vi "Read from File.vi"(7 "Section Name":string, 8 "error in (no error)":errorcluster, 10 "INI Ref":T1, 11 "Image Assertion in":refnum<class "Image Assertion.lvclass">) -> (0 "error out":errorcluster, 2 "INI Ref out":T1, 3 "Image Assertion out":refnum<class "Image Assertion.lvclass">)   [LabVIEW 2020, in "MacroAssert.lvlib" / "Image Assertion.lvclass"]
doc: "Reads associated parameters from the file identified by <B>INI Ref</B>."
uses:
  Image Assertion.lvclass
  <vilib>/Utility/config.llb/Config Data RefNum.ctl
  Image Assertion Type.ctl
  Image Comparator.ctl
  Image Units.ctl
  Compare Method.ctl
  <vilib>/picture/picture.llb/imagedata.ctl
  <vilib>/Utility/error.llb/Error Cluster From Error Code.vi
  <vilib>/Utility/config.llb/Read Key (String).vi
  <vilib>/Utility/config.llb/Read Key (I32).vi
  <vilib>/Utility/config.llb/Read Key (Double).vi
  Assertion Step/Assertion Step.lvclass
  SubVIs/Custom Errors/Custom Errors.lvlib
  <vilib>/Utility/config.llb/NI_LVConfig.lvlib
  MacroAssert.lvlib
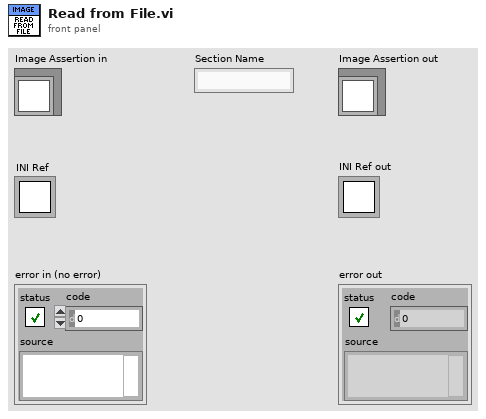
[diagram p1: front panel]
types:
  T1 = typedef "NI_LVConfig.lvlib/Config Data RefNum.ctl" = refnum<k1>
  T2 = typedef "MacroAssert.lvlib/Image Assertion.lvclass/Image Assertion Type.ctl" = enum16{"Control Image", "VI Image", "Window Image", "Cursor Icon"}
  T3 = typedef "MacroAssert.lvlib/Image Assertion.lvclass/Image Comparator.ctl" = enum16{"Is less than or equal to", "Is greater than or equal to"}
  T4 = typedef "MacroAssert.lvlib/Image Assertion.lvclass/Image Units.ctl" = enum16{"Pixels", "Percent"}
  T5 = typedef "MacroAssert.lvlib/Image Assertion.lvclass/Compare Method.ctl" = enum16{"Mean Squared Error", "Peak Signal-to-Noise Ratio"}
  T6 = typedef "imagedata.ctl" = cluster{"image type":i32, "image depth":i32, "image":u8[], "mask":u8[], "colors":u32[], "Rectangle":cluster{"left":i16, "top":i16, "right":i16, "bottom":i16}}
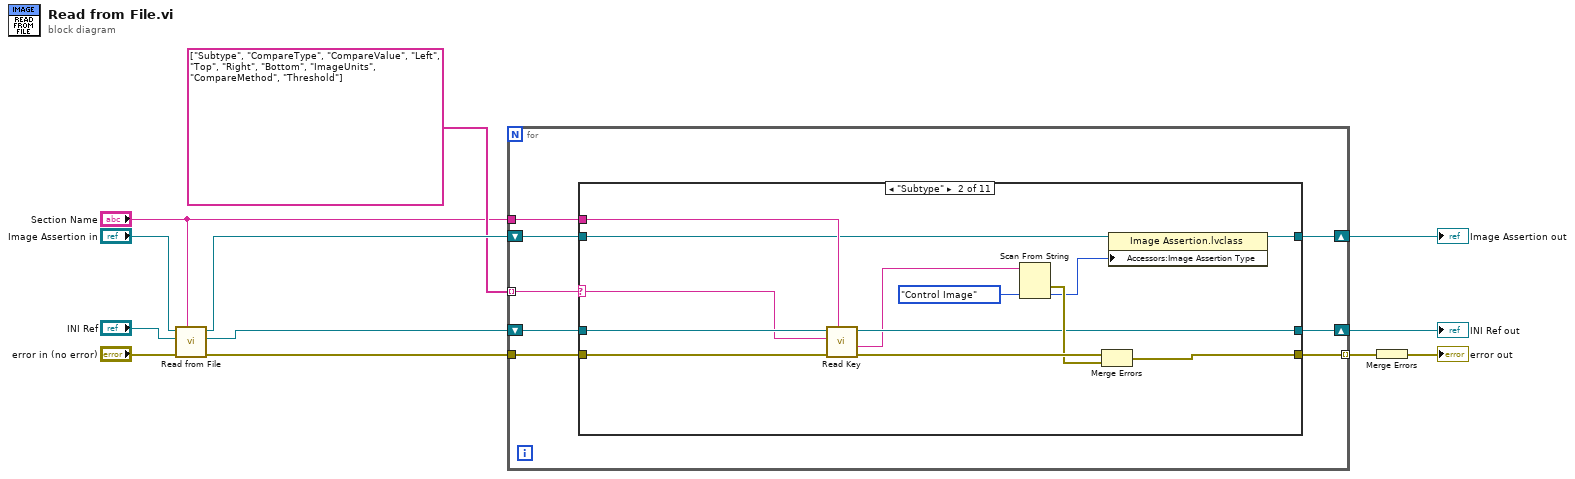
[diagram p0: block diagram]
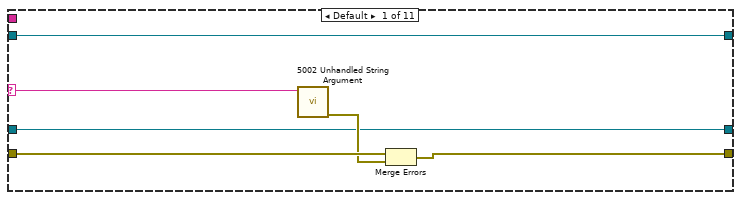
[diagram p2: hidden frame]
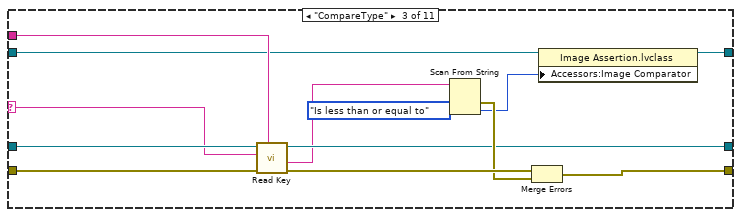
[diagram p3: hidden frame]
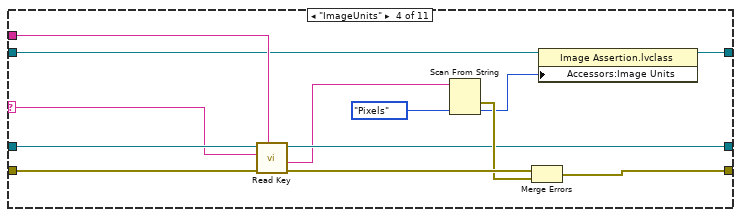
[diagram p4: hidden frame]
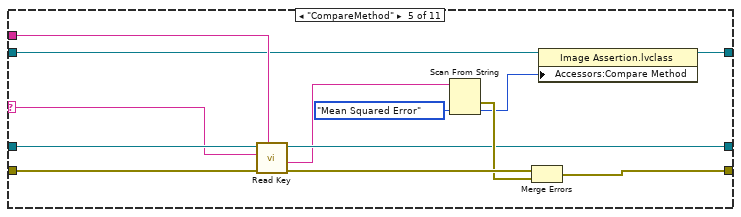
[diagram p5: hidden frame]
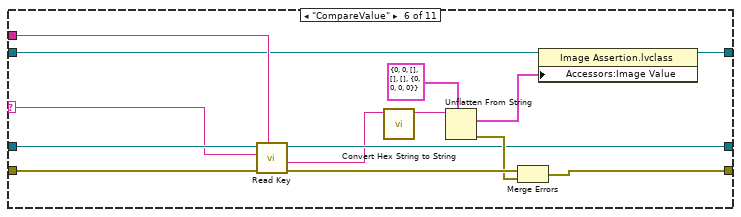
[diagram p6: hidden frame]
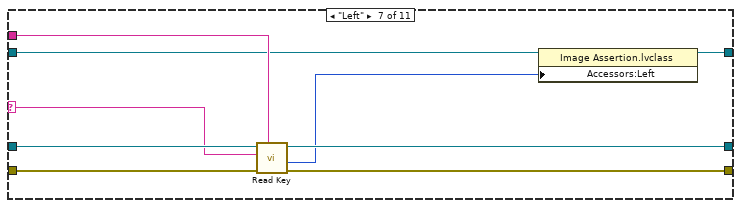
[diagram p7: hidden frame]
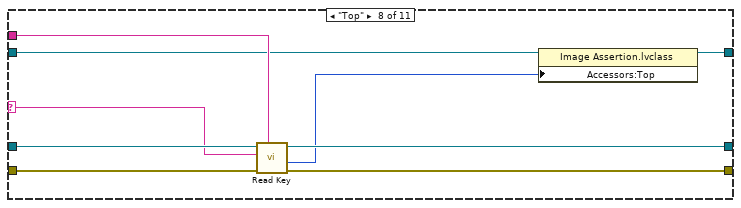
[diagram p8: hidden frame]
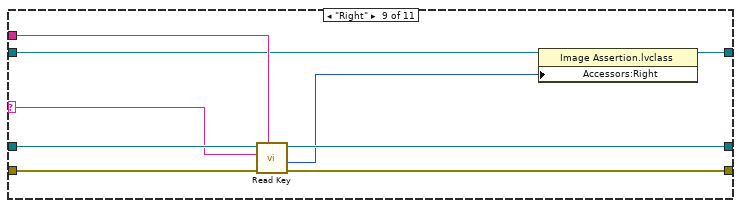
[diagram p9: hidden frame]
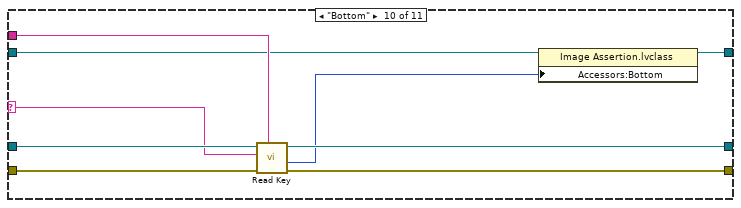
[diagram p10: hidden frame]
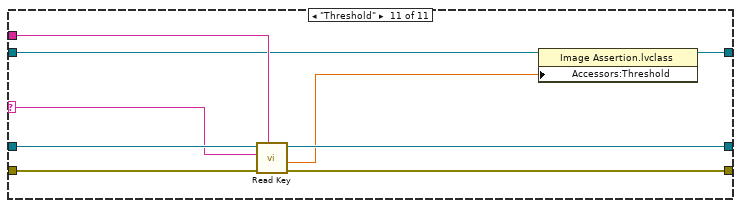
[diagram p11: hidden frame]
diagram:
  n1 = call-parent "Read from File.vi"("Section Name"="Section Name", "error in (no error)"="error in (no error)", "INI Ref"="INI Ref", "Assertion Step in"="Image Assertion in") -> ("error out"=w12:errorcluster, "INI Ref out"=w9:T1, "Assertion Step out"=w6:refnum<class "Image Assertion.lvclass">)  [unwired: 5 in]
  n2 = for {
    tunnel: string[] ["Subtype", "CompareType", "CompareValue", "Left", "Top", "Right", "Bottom", "ImageUnits", "CompareMethod", "Threshold"] -> [w16] mode=indexing
    tunnel: w12 -> [w20]
    tunnel: "Section Name" -> [w15]
    shift-right: [w13] -> w2
    shift-left: w6 -> [w14]
    tunnel: [w19] -> w4 mode=indexing
    shift-right: [w17] -> w7
    shift-left: w9 -> [w18]
    n3 = case shown="\"Subtype\"" w16 {
      selector: w16 -> [w21 w30 w43 w56 w69 w83 w94 w103 w112 w121 w130]
      tunnel: w20 -> [w26 w39 w52 w65 w78 w92 w101 w110 w119 w128 w137]
      tunnel: w15 -> [_ w33 w46 w59 w72 w86 w97 w106 w115 w124 w133]
      tunnel: w14 -> [w22 w32 w45 w58 w71 w85 w96 w105 w114 w123 w132]
      tunnel: [w22 w31 w44 w57 w70 w84 w95 w104 w113 w122 w131] -> w13
      tunnel: [w24 w37 w50 w63 w76 w89 w100 w109 w118 w127 w136] -> w19
      tunnel: w18 -> [w23 w35 w48 w61 w74 w88 w99 w108 w117 w126 w135]
      tunnel: [w23 w34 w47 w60 w73 w87 w98 w107 w116 w125 w134] -> w17
      frame Default {
        n4 = call "5002 Unhandled String Argument.vi"("Argument"=w21) -> ("error out"=w25:errorcluster)  [unwired: 10 in]
        n5 = Merge Errors(w26, w25) -> (w24:errorcluster)
      }
      frame "Subtype" {
        n6 = call-poly <vilib>:"Read Key.vi"("section"=w33, "error in (no error)"=w39, "key"=w30, "refnum"=w35) -> ("error out"=w38:errorcluster, "value"=w29:string, "refnum out"=w34:T1)  [unwired: 4 in, 1 out]
        n7 = Scan From String(input string=w29, default 1=Image_Assertion_Type."Control Image" ("Image Assertion Type")) -> (error out=w36:errorcluster, output 1=w28:T2)  [unwired: 3 in, 2 out]
        n8 = Merge Errors(w38, w36) -> (w37:errorcluster)
        n9 = property class="Image Assertion.lvclass"(reference=w32, "Accessors:Image Assertion Type"=w28) -> (reference out=w31:refnum<class "Image Assertion.lvclass">)  [unwired: 1 in, 1 out]
      }
      frame "CompareType" {
        n10 = call-poly <vilib>:"Read Key.vi"("section"=w46, "error in (no error)"=w52, "key"=w43, "refnum"=w48) -> ("error out"=w51:errorcluster, "value"=w42:string, "refnum out"=w47:T1)  [unwired: 4 in, 1 out]
        n11 = Scan From String(input string=w42, default 1=Image_Comparator."Is less than or equal to" ("Image Comparator")) -> (error out=w49:errorcluster, output 1=w41:T3)  [unwired: 3 in, 2 out]
        n12 = Merge Errors(w51, w49) -> (w50:errorcluster)
        n13 = property class="Image Assertion.lvclass"(reference=w45, "Accessors:Image Comparator"=w41) -> (reference out=w44:refnum<class "Image Assertion.lvclass">)  [unwired: 1 in, 1 out]
      }
      frame "ImageUnits" {
        n14 = call-poly <vilib>:"Read Key.vi"("section"=w59, "error in (no error)"=w65, "key"=w56, "refnum"=w61) -> ("error out"=w64:errorcluster, "value"=w55:string, "refnum out"=w60:T1)  [unwired: 4 in, 1 out]
        n15 = Scan From String(input string=w55, default 1=Image_Units."Pixels" ("Image Units")) -> (error out=w62:errorcluster, output 1=w54:T4)  [unwired: 3 in, 2 out]
        n16 = Merge Errors(w64, w62) -> (w63:errorcluster)
        n17 = property class="Image Assertion.lvclass"(reference=w58, "Accessors:Image Units"=w54) -> (reference out=w57:refnum<class "Image Assertion.lvclass">)  [unwired: 1 in, 1 out]
      }
      frame "CompareMethod" {
        n18 = call-poly <vilib>:"Read Key.vi"("section"=w72, "error in (no error)"=w78, "key"=w69, "refnum"=w74) -> ("error out"=w77:errorcluster, "value"=w68:string, "refnum out"=w73:T1)  [unwired: 4 in, 1 out]
        n19 = Scan From String(input string=w68, default 1=Compare_Method."Mean Squared Error" ("Compare Method")) -> (error out=w75:errorcluster, output 1=w67:T5)  [unwired: 3 in, 2 out]
        n20 = Merge Errors(w77, w75) -> (w76:errorcluster)
        n21 = property class="Image Assertion.lvclass"(reference=w71, "Accessors:Compare Method"=w67) -> (reference out=w70:refnum<class "Image Assertion.lvclass">)  [unwired: 1 in, 1 out]
      }
      frame "CompareValue" {
        n22 = call-poly <vilib>:"Read Key.vi"("section"=w86, "error in (no error)"=w92, "key"=w83, "refnum"=w88) -> ("error out"=w91:errorcluster, "value"=w80:string, "refnum out"=w87:T1)  [unwired: 4 in, 1 out]
        n23 = call "Convert Hex String to String.vi"("Hex String"=w80) -> ("String"=w79:string)  [unwired: 10 in]
        n24 = Unflatten From String(type=T6 {"image type"=0, "image depth"=0, "image"=[], "mask"=[], "colors"=[], "Rectangle"={"left"=0, "top"=0, "right"=0, "bottom"=0}} ("Expected Image"), binary string=w79) -> (value=w81:T6, error out=w90:errorcluster)  [unwired: 3 in, 1 out]
        n25 = Merge Errors(w91, w90) -> (w89:errorcluster)
        n26 = property class="Image Assertion.lvclass"(reference=w85, "Accessors:Image Value"=w81) -> (reference out=w84:refnum<class "Image Assertion.lvclass">)  [unwired: 1 in, 1 out]
      }
      frame "Left" {
        n27 = call-poly <vilib>:"Read Key.vi"("section"=w97, "error in (no error)"=w101, "key"=w94, "refnum"=w99) -> ("error out"=w100:errorcluster, "value"=w93:i32, "refnum out"=w98:T1)  [unwired: 4 in, 1 out]
        n28 = property class="Image Assertion.lvclass"(reference=w96, "Accessors:Left"=w93) -> (reference out=w95:refnum<class "Image Assertion.lvclass">)  [unwired: 1 in, 1 out]
      }
      frame "Top" {
        n29 = call-poly <vilib>:"Read Key.vi"("section"=w106, "error in (no error)"=w110, "key"=w103, "refnum"=w108) -> ("error out"=w109:errorcluster, "value"=w102:i32, "refnum out"=w107:T1)  [unwired: 4 in, 1 out]
        n30 = property class="Image Assertion.lvclass"(reference=w105, "Accessors:Top"=w102) -> (reference out=w104:refnum<class "Image Assertion.lvclass">)  [unwired: 1 in, 1 out]
      }
      frame "Right" {
        n31 = call-poly <vilib>:"Read Key.vi"("section"=w115, "error in (no error)"=w119, "key"=w112, "refnum"=w117) -> ("error out"=w118:errorcluster, "value"=w111:i32, "refnum out"=w116:T1)  [unwired: 4 in, 1 out]
        n32 = property class="Image Assertion.lvclass"(reference=w114, "Accessors:Right"=w111) -> (reference out=w113:refnum<class "Image Assertion.lvclass">)  [unwired: 1 in, 1 out]
      }
      frame "Bottom" {
        n33 = call-poly <vilib>:"Read Key.vi"("section"=w124, "error in (no error)"=w128, "key"=w121, "refnum"=w126) -> ("error out"=w127:errorcluster, "value"=w120:i32, "refnum out"=w125:T1)  [unwired: 4 in, 1 out]
        n34 = property class="Image Assertion.lvclass"(reference=w123, "Accessors:Bottom"=w120) -> (reference out=w122:refnum<class "Image Assertion.lvclass">)  [unwired: 1 in, 1 out]
      }
      frame "Threshold" {
        n35 = call-poly <vilib>:"Read Key.vi"("section"=w133, "error in (no error)"=w137, "key"=w130, "refnum"=w135) -> ("error out"=w136:errorcluster, "value"=w129:dbl, "refnum out"=w134:T1)  [unwired: 4 in, 1 out]
        n36 = property class="Image Assertion.lvclass"(reference=w132, "Accessors:Threshold"=w129) -> (reference out=w131:refnum<class "Image Assertion.lvclass">)  [unwired: 1 in, 1 out]
      }
    }
  }
  "Image Assertion out" <- w2
  "INI Ref out" <- w7
  n37 = Merge Errors(w4) -> (→"error out":errorcluster)
